vi "Debug.vi"(8 "error in (no error)":errorcluster, 9 "Numeric 1":dbl=nan, 10 "Numeric 0":dbl=nan, 11 "Heater in":refnum<class "Heater.lvclass">) -> (0 "error out":errorcluster, 3 "Heater out":refnum<class "Heater.lvclass">)   [LabVIEW 2015, in "cRIO-Carbondioxide.lvlib" / "CO2-Actor.lvlib" / "Heater.lvclass"]
uses:
  Heater.lvclass
  CO2 Actor/CO2 Actor.lvclass
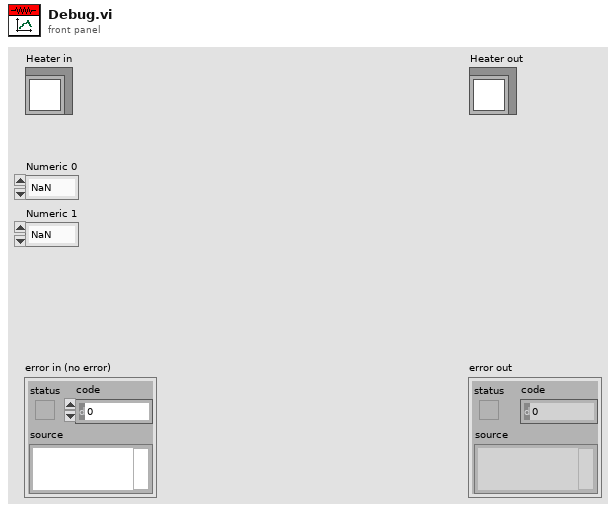
[diagram p1: front panel]
types:
  T1 = cluster{"Numeric 0":dbl, "Numeric 1":dbl, "Numeric 2":dbl, "Numeric 3":dbl, "Numeric 4":dbl, "Numeric 5":dbl, "Numeric 6":dbl, "Numeric 7":dbl}
  T2 = typedef "cRIO-Carbondioxide.lvlib/cRIO-CO2.lvlib/cRIO-CO2.lvclass/Debugger.ctl" = cluster{"Log Ref":refnum<vi>, "Debugger Graph Chart Ref":refnum<vi>, "Debug Rng Ref":refnum<vi>}
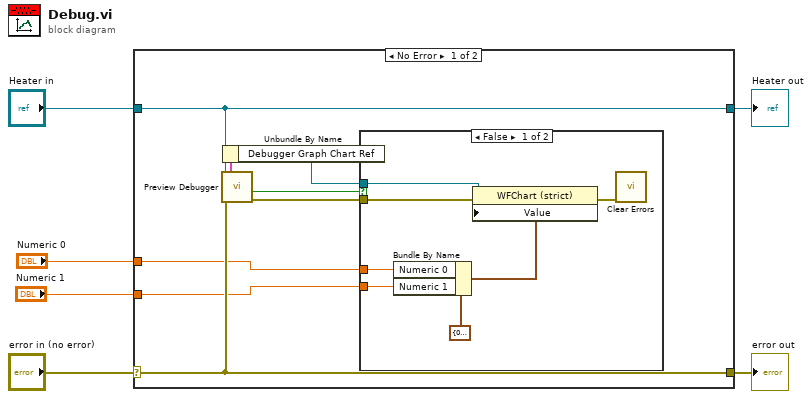
[diagram p0: block diagram]
diagram:
  n1 = case shown="No Error" "error in (no error)" {
    selector: "error in (no error)" -> [w13 w23]
    tunnel: [w13 w23] -> w5
    tunnel: [w9 w22] -> w3
    tunnel: "Heater in" -> [w9 w22]
    tunnel: "Numeric 0" -> [w11 _]
    tunnel: "Numeric 1" -> [w10 _]
    frame No Error {
      n2 = call "Preview Debugger.vi"("error in (no error)"=w13, "CO2 Actor in"=w9) -> ("error out"=w12:errorcluster, "timed out?"=w14:bool, "Debugger"=w8:T2)  [unwired: 6 in, 1 out]
      n3 = Unbundle By Name(w8) -> ("Debugger Graph Chart Ref"=w7:refnum<vi>)
      n4 = case shown="False" w14 {
        tunnel: w12 -> [w20 _]
        tunnel: w7 -> [w21 _]
        tunnel: w11 -> [w19 _]
        tunnel: w10 -> [w18 _]
        frame False {
          n5 = Bundle By Name(cluster=T1 {"Numeric 0"=0.0, "Numeric 1"=0.0, "Numeric 2"=nan, "Numeric 3"=nan, "Numeric 4"=nan, "Numeric 5"=nan, "Numeric 6"=nan, "Numeric 7"=nan} ("Debugger Graph Chart"), "Numeric 0"=w19, "Numeric 1"=w18) -> (w16:T1)
          n6 = property class="WFChart (strict)"(reference=w21, error in=w20, "Value"=w16) -> (error out=w17:errorcluster)  [unwired: 1 out]
          n7 = call <vilib>:"Clear Errors.vi"("error in (no error)"=w17) -> ()  [unwired: 5 in, 2 out]
        }
        frame True {
        }
      }
    }
    frame Error {
    }
  }
  "error out" <- w5
  "Heater out" <- w3
